vi "OS_ExecuteCmd.vi"(7 "wait until completion? (T)":bool=TRUE, 8 "error in (no error)":errorcluster, 9 "Comment":string, 10 "Command":string, 11 "Arduino In":T1) -> (0 "error out":errorcluster, 3 "Arduino out":T1)   [LabVIEW 2020]
uses:
  Arduino.ctl
panel:
  out "Console":string
  # "/private/var/folders/94/c619kr_57q99r5k1n1y2y_g40000gn/T/TemporaryItems/Arduino"
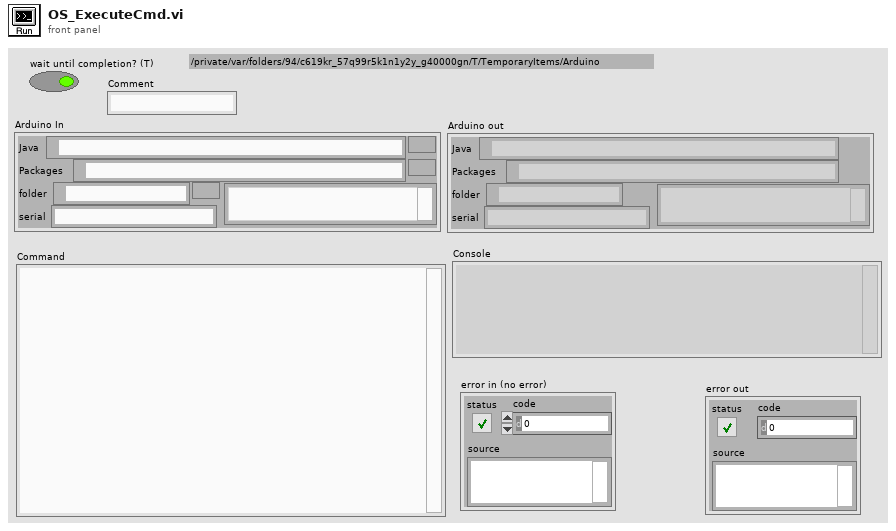
[diagram p1: front panel]
types:
  T1 = typedef "Arduino.ctl" = cluster{"Java":path, "Packages":path, "folder":path, "serial":string, "Console":string}
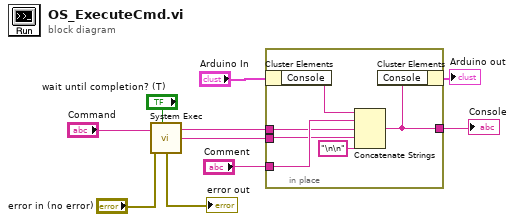
[diagram p0: block diagram]
diagram:
  n1 = call <vilib>:"System Exec.vi"("wait until completion? (T)"="wait until completion? (T)", "error in (no error)"="error in (no error)", "command line"="Command") -> ("error out"=→"error out":errorcluster, "standard error"=w3:string, "standard output"=w2:string)  [unwired: 5 in, 1 out]
  n2 = in-place {
    in-place-border: "Comment" -> [w16]
    in-place-border: w3 -> [w13]
    in-place-border: w2 -> [w12]
    in-place-border: [w11] -> w1
    n3 = in-place-cluster #1("Arduino In") -> ("Console"=w14:string)
    n4 = Concatenate Strings(w14, w16, w12, w13, "\n\n" ("string")) -> (w11:string)
    n5 = in-place-cluster #1("Console"=w11) -> (→"Arduino out":T1)
  }
  "Console" <- w1
